vi "Get SLSC Switch Model.vi"(8 "error in (no error)":errorcluster, 11 "SLSC Switch Custom Device Ref in":T1 format="%.0x") -> (0 "error out":errorcluster, 2 "Model":string, 3 "SLSC Switch Custom Device Ref out":T1 format="%.0x")   [LabVIEW 2017, in "SLSC Switch Scripting.lvlib"]
uses:
  SLSC Switch Scripting.lvlib
  <vilib>/NI Veristand/Custom Device API/Custom Device Item Ref.ctl
  SLSC Scripting Constants.vi
  Shared/Constants.vi
  <vilib>/NI Veristand/Custom Device API/Get Item Property (String).vi
  <vilib>/NI VeriStand/Custom Device API/Custom Device API.lvlib
  Shared/SLSC Switch Shared.lvlib
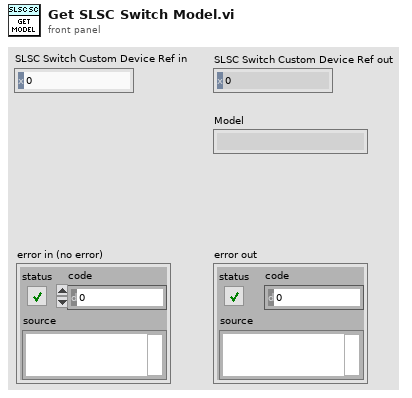
[diagram p1: front panel]
types:
  T1 = typedef "Custom Device API.lvlib/Custom Device Item Ref.ctl" = u64
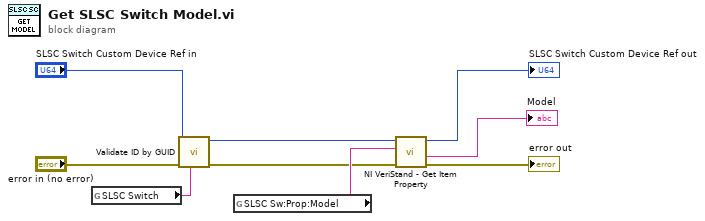
[diagram p0: block diagram]
diagram:
  n1 = global read "Constants.vi" "SLSC Switch"() -> (w1:string)
  n2 = call "Validate ID by GUID.vi"("GUID"=w1, "error in (no error)"="error in (no error)", "Ref ID in"="SLSC Switch Custom Device Ref in") -> ("error out"=w4:errorcluster, "Ref ID out"=w2:T1)  [unwired: 7 in]
  n3 = global read "SLSC Scripting Constants.vi" "SLSC Sw:Prop:Model"() -> (w7:string)
  n4 = call-poly <vilib>:"NI VeriStand - Get Item Property.vi"("error in (no error)"=w4, "Property Name"=w7, "Item Ref in"=w2) -> ("error out"=→"error out":errorcluster, "Value"=→"Model":string, "Item Ref out"=→"SLSC Switch Custom Device Ref out":T1)  [unwired: 5 in, 1 out]
